vi "Read Algae Operation.vi"(8 "Command Info":T4) -> (0 "Command Info":T4, 1 "SubSystem Data":T1={"Operation"=enum."Reserve", "Setpoint"=0.0, "Duration"=0.0, "Algae State"=enum."Intake Algae", "Negate or Confirm?"=FALSE}, 2 "Command Timing":cluster{"Start Time (ms)":u32, "Iterations":i32})   [LabVIEW 2023]
doc: "This returns the most recently scheduled command. This doesn't indicate whether the command finished and is running the default command."
uses:
  <vilib>/Rock Robotics/WPI/Framework/Command Status Info.ctl
  <vilib>/Rock Robotics/WPI/Framework/Completion Status.ctl
  <vilib>/Rock Robotics/WPI/Framework/Completion Notifier.ctl
  Implementation/Algae Setpoints.ctl
  Implementation/Algae Operations.ctl
  Support Code/Teleop Util/Algae States.ctl
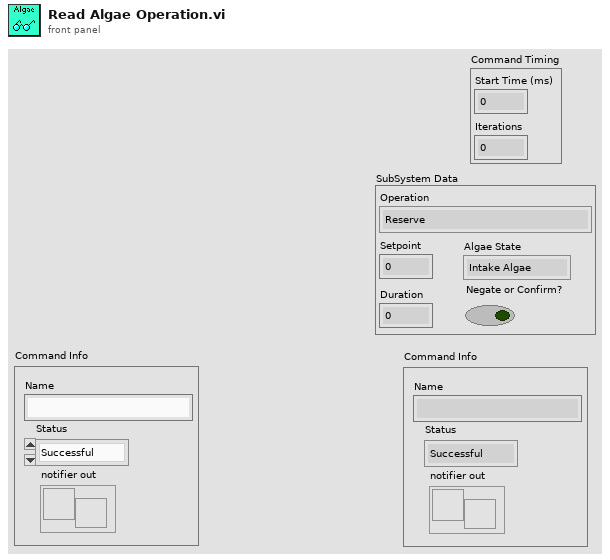
[diagram p1: front panel]
types:
  T1 = typedef "Algae Setpoints.ctl" = cluster{"Operation":T2, "Setpoint":dbl, "Duration":dbl, "Algae State":T3, "Negate or Confirm?":bool}
  T2 = typedef "Algae Operations.ctl" = enum16{"Reserve", "Read Current", "Immediate", "Calibrate"}
  T3 = typedef "Algae States.ctl" = enum16{"Idle", "Intake Algae", "Outtake Algae", "Stow", "Manual Overrides"}
  T4 = typedef "Command Status Info.ctl" = cluster{"Name":string, "Status":T5, "notifier out":T6}
  T5 = typedef "Completion Status.ctl" = enum16{"Successful", "Aborted", "Incomplete"}
  T6 = typedef "Completion Notifier.ctl" = refnum<notifier>
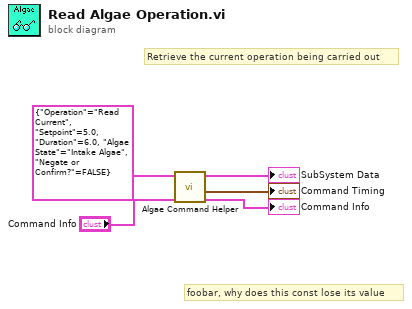
[diagram p0: block diagram]
diagram:
  # "foobar, why does this const lose its value"
  # "Retrieve the current operation being carried out"
  n1 = call "Algae Command Helper.vi"("Command Info In"="Command Info", "SubSystem Data"=T1 {"Operation"=enum."Read Current", "Setpoint"=5.0, "Duration"=6.0, "Algae State"=enum."Intake Algae", "Negate or Confirm?"=FALSE}) -> ("Command Info Out"=→"Command Info":T4, "Command Timing"=→"Command Timing":cluster{"Start Time (ms)":u32, "Iterations":i32}, "SubSystem Data"=→"SubSystem Data":T1)  [unwired: 7 in]
